vi "Test.vi"() -> ()   [LabVIEW 2020]
uses:
  <vilib>/numeric/Random Number (Range) I64.vi
  <vilib>/Analysis/baseanly.llb/Mean (DBL).vi
  <vilib>/numeric/sub_Random U32.vi
  Classes/KD Tree Double/KD Tree Double.lvclass
  E:/Labview/LV 2020/Libs/flann/flann/Classes/KD Tree/KD Tree.lvclass
  Classes/KD Tree Double/Create KD Tree Double.vi
  Classes/KD Tree Double/Find Nearest Neighbors Index Double.vi
  Classes/KD Tree Double/Radius Search Double.vi
  Classes/KD Tree/KD Tree.lvclass
  <vilib>/Analysis/NI_AALBase.lvlib
  E:/Labview/LV 2020/Libs/flann/flann/Classes/KD Tree Double/KD Tree Double.lvclass
panel:
  out "x/y":dbl
  out "mean":dbl format="%0.2f"
  out "P4":dbl[][](array[numeric])
  out "Array":dbl[](array[numeric])
  out "Histogram Graph":T1(graph)
  out "P1":dbl[][](array[numeric])
  out "P2":dbl[][](array[numeric])
  out "Intensity Graph":dbl[][](graph)
  out "error out":errorcluster
  out "N Found":i32[](array[numeric])
  out "Dists 2":dbl[][](array[numeric])
  out "Indices 2":i32[][](array[numeric])
  out "Dists":dbl[][](array[numeric])
  out "Indices":i32[][](array[numeric])
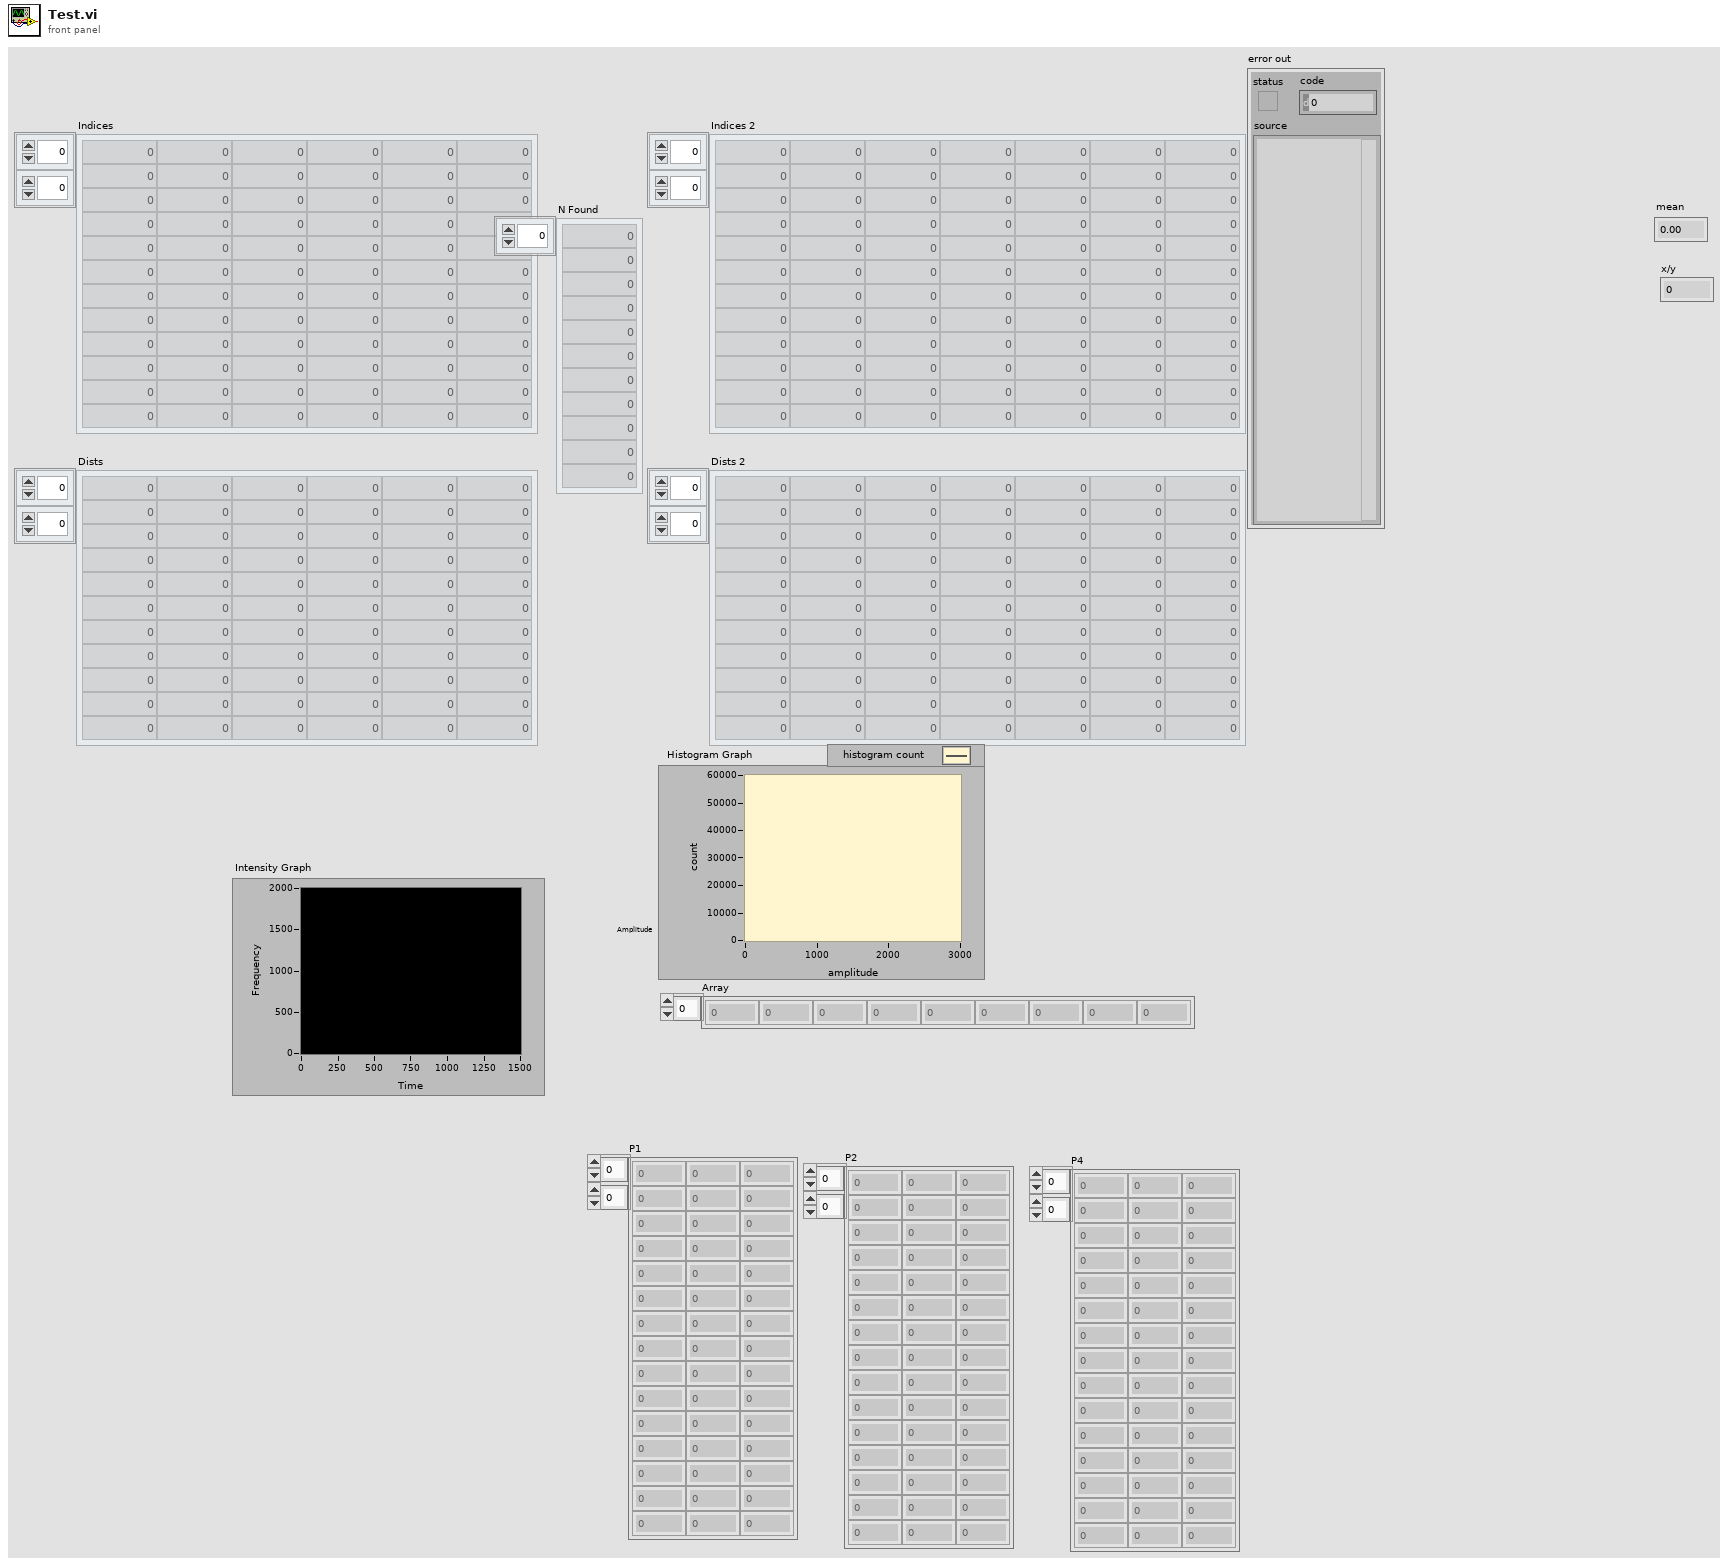
[diagram p1: front panel]
types:
  T1 = cluster{"X Values":dbl[], "Histogram: h(x)":i32[]}
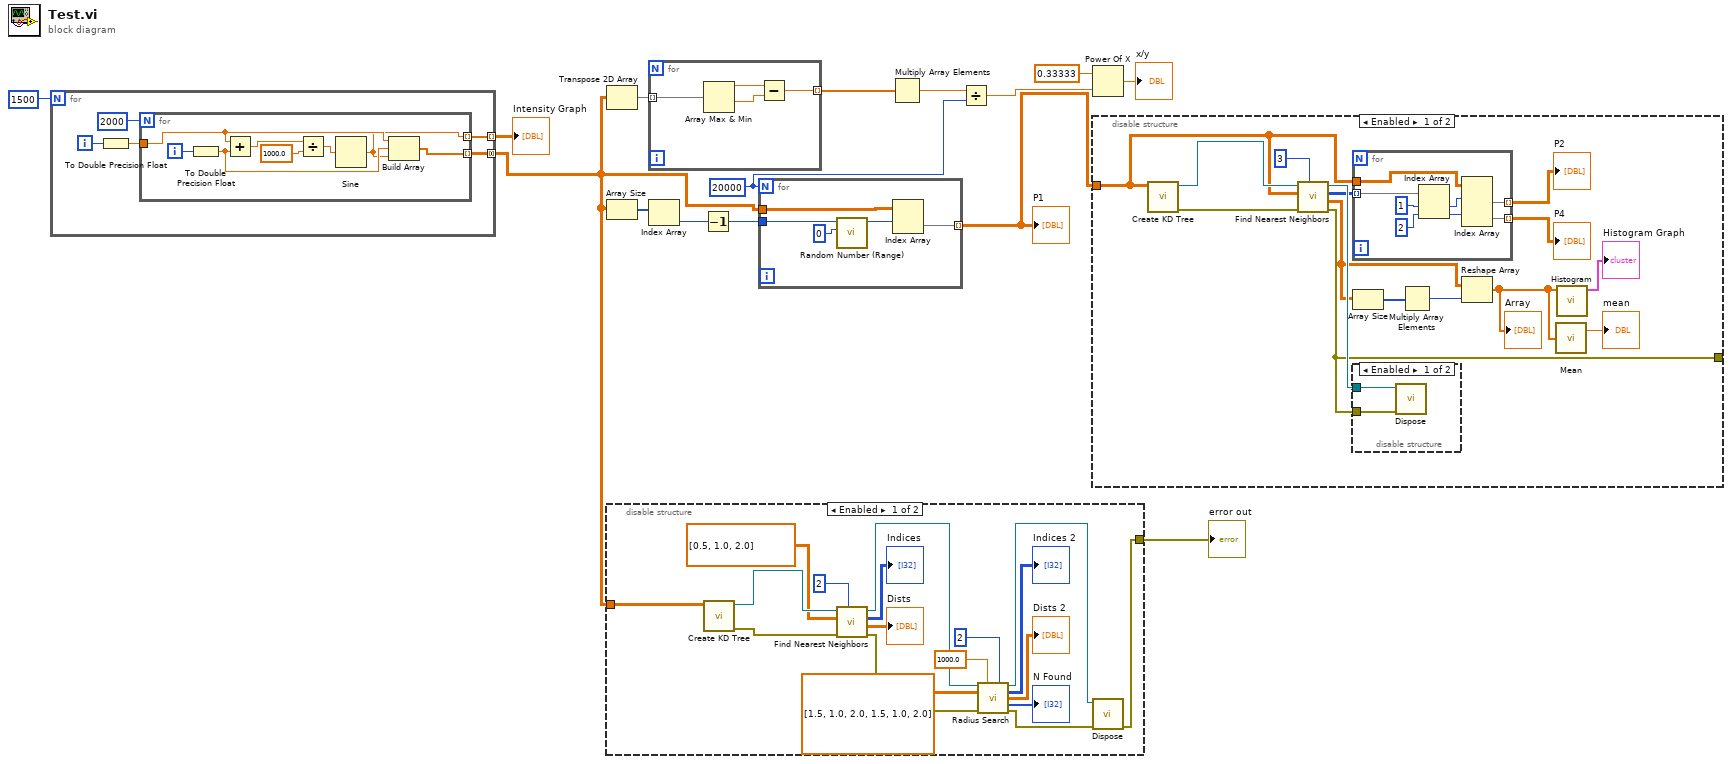
[diagram p0: block diagram]
diagram:
  w4 = 20000
  n1 = for {
    N: 1500 -> [_]
    tunnel: [w20] -> w8 mode=concatenating
    tunnel: [w16] -> w11 mode=indexing
    i -> [w19]
    n2 = To Double Precision Float(number=w19) -> (double precision float=w17:dbl)
    n3 = for {
      N: 2000 -> [_]
      tunnel: [w21] -> w20 mode=indexing
      tunnel: w17 -> [w26]
      tunnel: [w24] -> w16 mode=indexing
      i -> [w28]
      n4 = To Double Precision Float(number=w28) -> (double precision float=w27:dbl)
      n5 = Add(x=w26, y=w27) -> (x+y=w25:dbl)
      n6 = Divide(x=w25, y=1000.0) -> (x/y=w23:dbl)
      n7 = Sine(x=w23) -> (sin(x)=w24:dbl)
      n8 = Build Array(w26, w27, w24) -> (w21:dbl[])
    }
  }
  "Intensity Graph" <- w11
  n9 = Transpose 2D Array(2D array=w8) -> (transposed array=w7:dbl[][])
  n10 = Array Size(array=w8) -> (size(s)=w13:i32[])
  n11 = disable-structure shown="Enabled" {
    disable-tunnel: [w41 _] -> w15
    disable-tunnel: w8 -> [w40 _]
    frame Enabled {
      n12 = call-poly "Create KD Tree.vi"("Points (Row-Vectors)"=w40) -> ("error out"=w38:errorcluster, "KD Tree Double out"=w33:refnum<class "KD Tree Double.lvclass">)  [unwired: 9 in]
      n13 = call-poly "Find Nearest Neighbors.vi"("#Neighbors"=2, "error in (no error)"=w38, "Points"=dbl[][] [[0.5, 1.0, 2.0]], "KD Tree Double in"=w33) -> ("error out"=w37:errorcluster, "Dists"=→"Dists":dbl[][], "Indices"=→"Indices":i32[][], "KD Tree Double out"=w34:refnum<class "KD Tree Double.lvclass">)  [unwired: 4 in]
      n14 = call-poly "Radius Search.vi"("KD Tree Double in"=w34, "Radius"=sgl 1000.0, "Max Neighbors"=2, "Points"=dbl[][] [[1.5, 1.0, 2.0], [1.5, 1.0, 2.0]], "error in (no error)"=w37) -> ("KD Tree Double out"=w43:refnum<class "KD Tree Double.lvclass">, "Indices"=→"Indices 2":i32[][], "Dists"=→"Dists 2":dbl[][], "N Found"=→"N Found":i32[], "error out"=w42:errorcluster)  [unwired: 6 in]
      n15 = call "Dispose.vi"("error in (no error)"=w42, "KD Tree in"=w43) -> ("error out"=w41:errorcluster)  [unwired: 9 in]
    }
    frame Disabled {
    }
  }
  "error out" <- w15
  n16 = for {
    tunnel: w7 -> [w50] mode=indexing
    tunnel: [w47] -> w6 mode=indexing
    n17 = Array Max & Min(array=w50) -> (max value=w49:dbl, min value=w48:dbl)  [unwired: 2 out]
    n18 = Subtract(x=w49, y=w48) -> (x-y=w47:dbl)
  }
  n19 = Index Array(array=w13) -> (element=w10:i32)  [unwired: 1 in]
  n20 = Decrement(x=w10) -> (x-1=w12:i32)
  n21 = for {
    N: w4 -> [_]
    tunnel: w8 -> [w55]
    tunnel: w12 -> [w53]
    tunnel: [w51] -> w9 mode=indexing
    n22 = call-poly <vilib>:"Random Number (Range).vi"("lower bound (-100)"=i64 0, "upper bound (100)"=w53) -> ("number"=w54:i64)  [unwired: 9 in]
    n23 = Index Array(array=w55, index (row)=w54) -> (element=w51:dbl[])  [unwired: 1 in]
  }
  "P1" <- w9
  n24 = Multiply Array Elements(1:w6) -> (0:w5:dbl)
  n25 = Divide(x=w5, y=w4) -> (x/y=w3:dbl)
  n26 = Power Of X(1:w3, 2:0.33333 ("x")) -> (0:→"x/y":dbl)
  n27 = disable-structure shown="Enabled" {
    disable-tunnel: w9 -> [w68 _]
    disable-tunnel: [w61 _] -> _
    frame Enabled {
      n28 = call-poly "Create KD Tree.vi"("Points (Row-Vectors)"=w68) -> ("error out"=w69:errorcluster, "KD Tree Double out"=w70:refnum<class "KD Tree Double.lvclass">)  [unwired: 9 in]
      n29 = call-poly "Find Nearest Neighbors.vi"("#Neighbors"=3, "error in (no error)"=w69, "Points"=w68, "KD Tree Double in"=w70) -> ("error out"=w61:errorcluster, "Dists"=w63:dbl[][], "Indices"=w60:i32[][], "KD Tree Double out"=w65:refnum<class "KD Tree Double.lvclass">)  [unwired: 4 in]
      n30 = for {
        tunnel: w68 -> [w80]
        tunnel: [w79] -> w67 mode=indexing
        tunnel: [w78] -> w66 mode=indexing
        tunnel: w60 -> [w77] mode=indexing
        n31 = Index Array(array=w77, index #1=1 ("disabled index (col)"), index #2=2 ("index (col)")) -> (element #1=w74:i32, element #2=w73:i32)
        n32 = Index Array(array=w80, index (row) #1=w74, index (row) #2=w73) -> (element #1=w79:dbl[], element #2=w78:dbl[])  [unwired: 2 in]
      }
      "P2" <- w67
      "P4" <- w66
      n33 = Array Size(array=w63) -> (size(s)=w64:i32[])
      n34 = disable-structure shown="Enabled" {
        disable-tunnel: w65 -> [w72 _]
        disable-tunnel: w61 -> [w71 _]
        frame Enabled {
          n35 = call "Dispose.vi"("error in (no error)"=w71, "KD Tree in"=w72) -> ()  [unwired: 9 in, 1 out]
        }
        frame Disabled {
        }
      }
      n36 = Multiply Array Elements(1:w64) -> (0:w62:i32)
      n37 = Reshape Array(w63, w62) -> (w56:dbl[])
      "Array" <- w56
      n38 = call-poly <vilib>:"Mean.vi"("X"=w56) -> ("mean"=→"mean":dbl)  [unwired: 1 out]
      n39 = call <vilib>:"Histogram.vi"("X"=w56) -> ("Histogram Graph"=→"Histogram Graph":T1)  [unwired: 7 in, 3 out]
    }
    frame Disabled {
    }
  }
